vi "AOConvert.vi"(10 "Voltage Range":dbl, 11 "Signal":i16[][](array[numeric])) -> (2 "Retract":dbl[](array[numeric]), 3 "Approach":dbl[](array[numeric]))   [LabVIEW 2016]
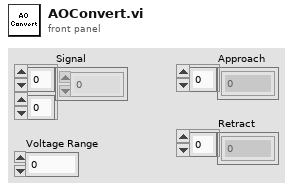
[diagram p1: front panel]
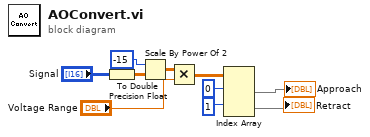
[diagram p0: block diagram]
diagram:
  n1 = To Double Precision Float(number="Signal") -> (double precision float=w2:dbl[][])
  n2 = Scale By Power Of 2(n=i16 -15, x=w2) -> (x*2^n=w8:dbl[][])
  n3 = Multiply(x=w8, y="Voltage Range") -> (x*y=w6:dbl[][])
  n4 = Index Array(array=w6, index (row) #1=0 ("index (row)"), index (row) #2=1 ("index (row)")) -> (element #1=→"Approach":dbl[], element #2=→"Retract":dbl[])  [unwired: 2 in]
